vi "Open DSI.vi"(8 "error in (no error)":errorcluster, 11 "DCM":refnum<class "DCM - RT.lvclass">) -> (0 "error out":errorcluster, 2 "Target Name":string, 3 "DSI Reference":refnum<class "DCM-DSI.lvclass">)   [LabVIEW 2016, in "DCM-DSI.lvclass"]
uses:
  DCM-DSI.lvclass
  <vilib>/Powertrain Controls/Device Drivers/DCM/Rev0/RT/DCM - RT.lvclass
  <vilib>/Powertrain Controls/Device Drivers/DCM/Diff IO/RT/Results.ctl
  <vilib>/Powertrain Controls/Device Drivers/DCM/HH/RT/Config.ctl
  <vilib>/Powertrain Controls/Device Drivers/DCM/HH/RT/Mode.ctl
  <vilib>/Powertrain Controls/Device Drivers/DCM/HH/RT/ISeq.ctl
  <vilib>/Powertrain Controls/Device Drivers/DCM/HH/RT/Status.ctl
  <vilib>/Powertrain Controls/Device Drivers/DCM/Rev0/RT/System State.ctl
  <vilib>/Powertrain Controls/Device Drivers/DCM/Rev0/RT/System ADC.ctl
  <vilib>/Powertrain Controls/Device Drivers/DCM/Rev0/RT/Internal Fault.ctl
  <vilib>/Powertrain Controls/Device Drivers/Engine Position Tracking/EPTx/RevA/RT/Controls/EPTxData.ctl
  Shared/Typedefs/Engine-Channel.ctl
  DCM-DSI.lvclass/DCM-DSI.ctl
  <vilib>/addons/Software Calibration Management/xSCM/CalPoint.xnode
  <vilib>/Powertrain Controls/Device Drivers/DCM/Diff IO/RT/DCM - RT - Diff IO.lvlib
  <vilib>/Powertrain Controls/Device Drivers/DCM/HH/RT/DCM - RT - HH.lvlib
  <vilib>/Powertrain Controls/Device Drivers/Engine Position Tracking/EPTx/RevA/RT/EPTx - RevA - RT.lvlib
  <resource>/objmgr/nisysapi.rc
  <vilib>/NI_Real-Time Target Support.lvlib
  <vilib>/addons/Software Calibration Management/xSCM/ni_scm.dll
  Shared/DSI-Shared.lvlib
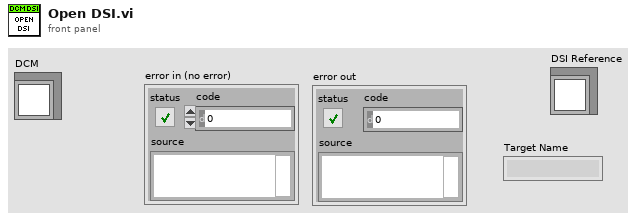
[diagram p1: front panel]
types:
  T1 = typedef "DSI-Shared.lvlib/Engine-Channel.ctl" = cluster{"Name":string, "Unit":string, "Value":sgl}
  T2 = typedef "EPTx - RevA - RT.lvlib/EPTxData.ctl" = cluster{"Sync":bool, "CurrentCAD":sgl, "Speed [RPM]":sgl, "Config":bool, "Rcvg Primary":bool, "Stall":bool, "Overflow":bool, "Ratio Error":bool, "Pattern Error":bool, "Aux Warning":bool, "Watchdog Error":bool}
  T3 = typedef "DCM - RT.lvclass/System State.ctl" = cluster{"System ADC":T4, "IO Lock":bool, "HH Mode Config Error":bool, "Fan Speed 1 [RPM]":sgl, "Fan Speed 2 [RPM]":sgl, "Firmware Major Rev":u16, "Firmware Minor Rev":u16, "Internal Fault":T5, "Fault Value":dbl}
  T4 = typedef "DCM - RT.lvclass/System ADC.ctl" = cluster{"AI 1 [V]":sgl, "AI 2 [V]":sgl, "AI 3 [V]":sgl, "AI 4 [V]":sgl, "AI 5 [V]":sgl, "AI 6 [V]":sgl, "AI 7 [V]":sgl, "AI 8 [V]":sgl, "AI 9 [V]":sgl, "AI 10 [V]":sgl, "AI 11 [V]":sgl, "AI 12 [V]":sgl, "Temp HH 1-6 [C]":sgl, "Temp HH 7-12 [C]":sgl, "Temp DI A [C]":sgl, "Temp DI Zener A [C]":sgl, "Temp DI B [C]":sgl, "Temp DI Zener B [C]":sgl, "Temp CPU [C]":sgl, "Temp Fan Intake [C]":sgl, "Temp Secondary A [C]":sgl, "Temp Primary A [C]":sgl, "Temp Boost B [C]":sgl, "Primary Range [V]":sgl, "Primary A1A2 [V]":sgl, "Primary A3A4 [V]":sgl, "Primary B3B4 [V]":sgl, "Primary B1B2 [V]":sgl, "Secondary A1A2 [V]":sgl, "Secondary A3A4 [V]":sgl, "Secondary B3B4 [V]":sgl, "Secondary B1B2 [V]":sgl, "Ext HV A [V]":sgl, "Ext HV B [V]":sgl, "FET Driver [V]":sgl, "Fan [V]":sgl, "Battery [V]":sgl, "DRVP [V]":sgl, "Key [V]":sgl, "DI Zener A [V]":sgl, "DI Zener B [V]":sgl, "Pump Zener A [V]":sgl, "Pump Zener B [V]":sgl, "MPRD [V]":sgl}
  T5 = typedef "DCM - RT.lvclass/Internal Fault.ctl" = enum32{"None", "Temp HH 1-6", "Temp HH 7-12", "Temp DI A", "Temp DI Zener A", "Temp DI B", "Temp DI Zener B", "Temp Intake", "Temp Primary A", "Temp Secondary A", "Temp Boost B", "Temp CPU", "Low Battery", "Inrush Protection", "A Run Enable", "B Run Enable", "Fan Speed"}
  T6 = typedef "DCM - RT - HH.lvlib/Status.ctl" = cluster{"Current [A]":sgl, "Config Error":bool, "Short Fault":bool, "Open Fault":bool, "Period Min [A]":sgl, "Period Max [A]":sgl, "Period Avg [A]":sgl, "On Avg [A]":sgl}
  T7 = typedef "DCM - RT - HH.lvlib/Config.ctl" = cluster{"Mode":T8, "IO Lock State":bool, "Phase 1 FP":bool, "Fault Clear":bool, "ISeq":T9[]}
  T8 = typedef "DCM - RT - HH.lvlib/Mode.ctl" = enum16{"Off", "Lowside", "Highside", "PFI", "Full H", "3-Phase"}
  T9 = typedef "DCM - RT - HH.lvlib/ISeq.ctl" = cluster{"Upper [A]":sgl, "Lower [A]":sgl, "Duration [s]":sgl}
  T10 = typedef "DCM - RT - Diff IO.lvlib/Results.ctl" = cluster{"Capture [DBTDC]":sgl, "Capture Error":bool, "Frequency [Hz]":sgl, "Duty Cycle [%]":sgl, "PWM Stopped":bool}
  T11 = cluster{"Mode":enum8{"Off", "Direct", "Calibration", "Triggered Multi-Pulse", "Engine Position Tracking"}, "Digital Input":enum8{"Unused", "User OS", "Diff IO 1", "Diff IO 2", "Diff IO 3", "Diff IO 4", "Diff IO 5", "Diff IO 6", "Diff IO 7", "Diff IO 8", "Aux 1", "Aux 2", "Aux 3", "Aux 4", "Aux 5", "Aux 6", "Aux 7", "Aux 8", "Aux 9", "Aux 10", "Aux 11", "Aux 12", "Aux 13", "Aux 14", "Aux 15", "Aux 16"}, "Default Profile Index":u8, "Cal Freq [Hz]":sgl, "Cal Duration [s]":sgl, "Cal Increment [s]":sgl, "Cal Pulses":u16, "TMP Command Sequence":cluster{"Duration [s]":sgl, "Level":bool, "Run/Stop":bool, "Profile Index":u8}[], "EPT TDC Offset [CAD]":sgl, "EPT Window Start [DBTDC]":sgl, "EPT Window End [DBTDC]":sgl, "EPT Angles":cluster{"Enable":bool, "Timing [DBTDC]":sgl, "Duration [s]":sgl, "Profile Index":u8}[], "EPT Skip Fire":bool, "EPT Skip Index":u8, "EPT Precharge Duration [s]":sgl, "EPT Precharge Profile Index":u8}[]
  T12 = cluster{"Mode":enum8{"Off", "Direct", "Calibration", "Triggered Multi-Pulse", "Engine Position Tracking"}, "Digital Input":enum8{"Unused", "User OS", "Diff IO 1", "Diff IO 2", "Diff IO 3", "Diff IO 4", "Diff IO 5", "Diff IO 6", "Diff IO 7", "Diff IO 8", "Aux 1", "Aux 2", "Aux 3", "Aux 4", "Aux 5", "Aux 6", "Aux 7", "Aux 8", "Aux 9", "Aux 10", "Aux 11", "Aux 12", "Aux 13", "Aux 14", "Aux 15", "Aux 16"}, "Default Profile Index":u8, "Cal Freq [Hz]":sgl, "Cal Duration [s]":sgl, "Cal Increment [s]":sgl, "Cal Pulses":u16, "TMP Command Sequence":cluster{"Duration [s]":sgl, "Level":bool, "Run/Stop":bool, "Profile Index":u8}[], "EPT TDC Offset [CAD]":sgl, "EPT Window Start [DBTDC]":sgl, "EPT Window End [DBTDC]":sgl, "EPT Angles":cluster{"Enable":bool, "Timing [DBTDC]":sgl, "Duration [s]":sgl, "Profile Index":u8}[], "EPT Skip Fire":bool, "EPT Skip Index":u8, "EPT Precharge Duration [s]":sgl, "EPT Precharge Profile Index":u8}
  T13 = cluster{"Mode":enum8{"Off", "Input", "Pulse Width Modulation", "Engine Position Tracking", "Serial Out 1", "Serial Out 2", "EPTx Sync"}, "Capture Start [DBTDC]":sgl, "Capture End [DBTDC]":sgl, "Invert":bool, "Frequency [Hz]":sgl, "Duty Cycle [%]":sgl, "TDC Offset [CAD]":sgl, "Window Start [DBTDC]":sgl, "Window End [DBTDC]":sgl, "Angles":cluster{"Enable":bool, "Location [DBTDC]":sgl, "Duration [s]":sgl}[], "Skip Fire":bool, "Skip Fire Index":u8}[]
  T14 = cluster{"Mode":enum8{"Off", "Direct", "Pulse Width Modulation", "Engine Position Tracking"}, "Digital Input":enum8{"Unused", "User OS", "Diff IO 1", "Diff IO 2", "Diff IO 3", "Diff IO 4", "Diff IO 5", "Diff IO 6", "Diff IO 7", "Diff IO 8", "Aux 1", "Aux 2", "Aux 3", "Aux 4", "Aux 5", "Aux 6", "Aux 7", "Aux 8", "Aux 9", "Aux 10", "Aux 11", "Aux 12", "Aux 13", "Aux 14", "Aux 15", "Aux 16"}, "Polarity":bool, "Frequency [Hz]":sgl, "Duty Cycle [%]":sgl, "TDC Offset [CAD]":sgl, "Window Start [DBTDC]":sgl, "Window End [DBTDC]":sgl, "Angles":cluster{"Enable":bool, "Location [DBTDC]":sgl, "Duration [s]":sgl}[], "Skip Fire":bool, "Skip Fire Index":u8}[]
  T15 = cluster{"Enable":bool, "Total Cycles":u8, "On Cycles":u8, "TDC Offset [CAD]":sgl}[]
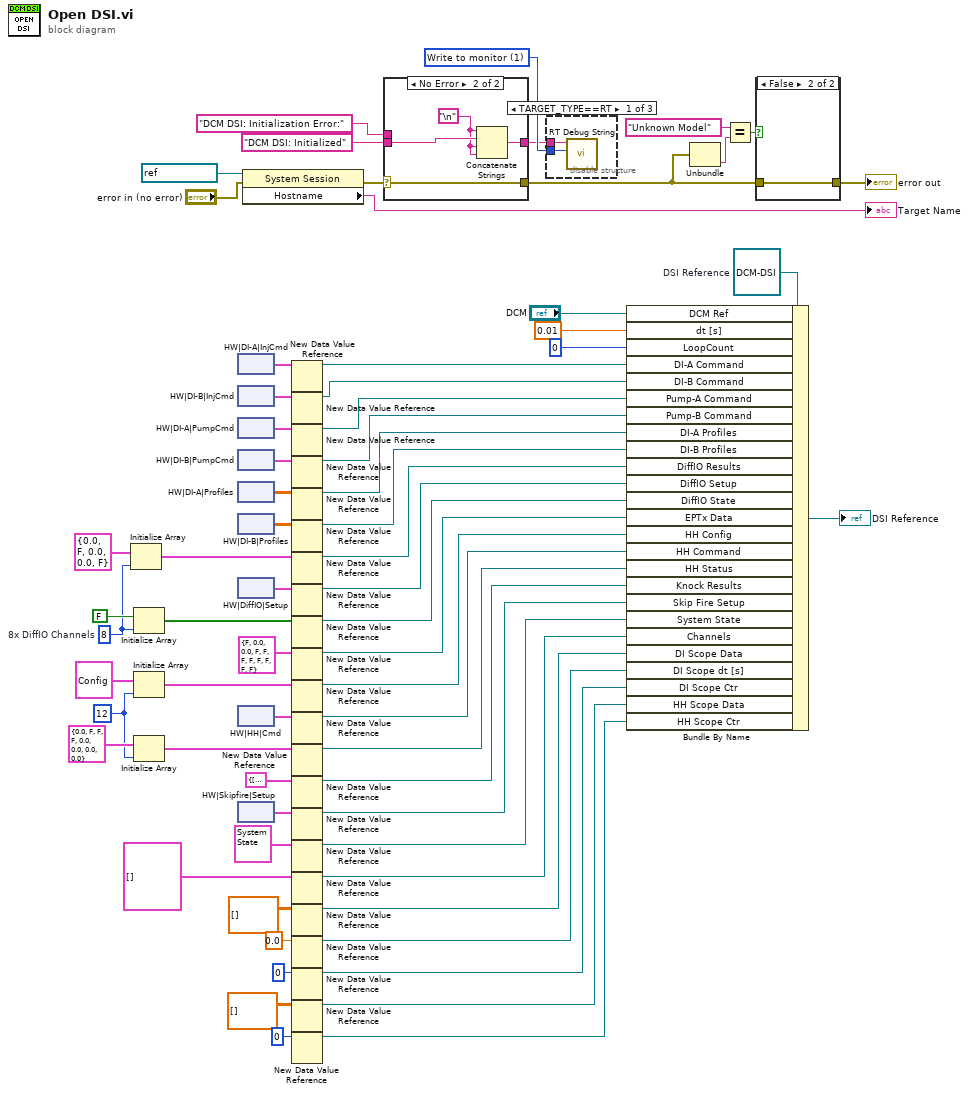
[diagram p0: block diagram]
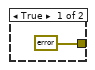
[diagram p4: hidden frame]
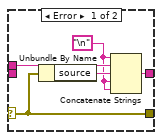
[diagram p5: hidden frame]
diagram:
  w10 = u16 1 items=["Write to serial", "Write to monitor", "Write to system log"] ("Interface")
  w56 = 12 ("dimension size")
  w19 = 8  # 8x DiffIO Channels
  w34 = refnum<class "DCM-DSI.lvclass"> refnum  # DSI Reference
  n1 = Initialize Array(T10 {"Capture [DBTDC]"=0.0, "Capture Error"=FALSE, "Frequency [Hz]"=0.0, "Duty Cycle [%]"=0.0, "PWM Stopped"=FALSE} ("Diff I/O Result"), w19) -> (w65:T10[])
  n2 = Initialize Array(FALSE ("Boolean"), w19) -> (w64:bool[])
  n3 = Initialize Array(T7 {"Mode"=enum."Off", "IO Lock State"=FALSE, "Phase 1 FP"=FALSE, "Fault Clear"=FALSE, "ISeq"=[{"Upper [A]"=0.0, "Lower [A]"=0.0, "Duration [s]"=0.0}, {"Upper [A]"=0.0, "Lower [A]"=0.0, "Duration [s]"=0.0}]} ("HH Config"), w56) -> (w62:T7[])
  n4 = Initialize Array(T6 {"Current [A]"=0.0, "Config Error"=FALSE, "Short Fault"=FALSE, "Open Fault"=FALSE, "Period Min [A]"=0.0, "Period Max [A]"=0.0, "Period Avg [A]"=0.0, "On Avg [A]"=0.0} ("HH Status"), w56) -> (w57:T6[])
  n5 = xnode "HW|DI-A|InjCmd"() -> ("Value"=w25:T11)
  n6 = xnode "HW|DI-B|InjCmd"() -> ("Value"=w23:T11)
  n7 = xnode "HW|DI-A|PumpCmd"() -> ("Value"=w24:T12)
  n8 = xnode "HW|DI-B|PumpCmd"() -> ("Value"=w22:T12)
  n9 = xnode "HW|DI-A|Profiles"() -> ("Value"=w21:sgl[][])
  n10 = xnode "HW|DI-B|Profiles"() -> ("Value"=w20:sgl[][])
  n11 = xnode "HW|DiffIO|Setup"() -> ("Value"=w17:T13)
  n12 = xnode "HW|HH|Cmd"() -> ("Value"=w16:T14)
  n13 = xnode "HW|Skipfire|Setup"() -> ("Value"=w15:T15)
  n14 = property class="System Session"(reference=refnum<k21> "localhost" ("Target (localhost)"), error in="error in (no error)") -> (error out=w1:errorcluster, "Hostname"=→"Target Name":string)  [unwired: 1 out]
  n15 = New Data Value Reference(data value=w25) -> (data value reference=w66:refnum<data-value>)  [unwired: 1 in, 1 out]
  n16 = New Data Value Reference(data value=w23) -> (data value reference=w26:refnum<data-value>)  [unwired: 1 in, 1 out]
  n17 = New Data Value Reference(data value=w24) -> (data value reference=w27:refnum<data-value>)  [unwired: 1 in, 1 out]
  n18 = New Data Value Reference(data value=w22) -> (data value reference=w28:refnum<data-value>)  [unwired: 1 in, 1 out]
  n19 = New Data Value Reference(data value=w21) -> (data value reference=w29:refnum<data-value>)  [unwired: 1 in, 1 out]
  n20 = New Data Value Reference(data value=w20) -> (data value reference=w30:refnum<data-value>)  [unwired: 1 in, 1 out]
  n21 = New Data Value Reference(data value=w65) -> (data value reference=w31:refnum<data-value>)  [unwired: 1 in, 1 out]
  n22 = New Data Value Reference(data value=w17) -> (data value reference=w18:refnum<data-value>)  [unwired: 1 in, 1 out]
  n23 = New Data Value Reference(data value=w64) -> (data value reference=w63:refnum<data-value>)  [unwired: 1 in, 1 out]
  n24 = New Data Value Reference(data value=T2 {"Sync"=FALSE, "CurrentCAD"=0.0, "Speed [RPM]"=0.0, "Config"=FALSE, "Rcvg Primary"=FALSE, "Stall"=FALSE, "Overflow"=FALSE, "Ratio Error"=FALSE, "Pattern Error"=FALSE, "Aux Warning"=FALSE, "Watchdog Error"=FALSE} ("HW.EPTxData")) -> (data value reference=w47:refnum<data-value>)  [unwired: 1 in, 1 out]
  n25 = New Data Value Reference(data value=w62) -> (data value reference=w60:refnum<data-value>)  [unwired: 1 in, 1 out]
  n26 = New Data Value Reference(data value=w16) -> (data value reference=w59:refnum<data-value>)  [unwired: 1 in, 1 out]
  n27 = New Data Value Reference(data value=w57) -> (data value reference=w55:refnum<data-value>)  [unwired: 1 in, 1 out]
  n28 = New Data Value Reference(data value=cluster{"Knock":bool[], "Knock Intensity":sgl[]} {"Knock"=[FALSE, FALSE, FALSE, FALSE, FALSE, FALSE, FALSE, FALSE, FALSE, FALSE, FALSE, FALSE, FALSE, FALSE, FALSE, FALSE], "Knock Intensity"=[0.0, 0.0, 0.0, 0.0, 0.0, 0.0, 0.0, 0.0, 0.0, 0.0, 0.0, 0.0, 0.0, 0.0, 0.0, 0.0]} ("HW.Knock Results")) -> (data value reference=w51:refnum<data-value>)  [unwired: 1 in, 1 out]
  n29 = New Data Value Reference(data value=w15) -> (data value reference=w54:refnum<data-value>)  [unwired: 1 in, 1 out]
  n30 = New Data Value Reference(data value=T3 {"System ADC"={"AI 1 [V]"=0.0, "AI 2 [V]"=0.0, "AI 3 [V]"=0.0, "AI 4 [V]"=0.0, "AI 5 [V]"=0.0, "AI 6 [V]"=0.0, "AI 7 [V]"=0.0, "AI 8 [V]"=0.0, "AI 9 [V]"=0.0, "AI 10 [V]"=0.0, "AI 11 [V]"=0.0, "AI 12 [V]"=0.0, "Temp HH 1-6 [C]"=0.0, "Temp HH 7-12 [C]"=0.0, "Temp DI A [C]"=0.0, "Temp DI Zener A [C]"=0.0, "Temp DI B [C]"=0.0, "Temp DI Zener B [C]"=0.0, "Temp CPU [C]"=0.0, "Temp Fan Intake [C]"=0.0, "Temp Secondary A [C]"=0.0, "Temp Primary A [C]"=0.0, "Temp Boost B [C]"=0.0, "Primary Range [V]"=0.0, "Primary A1A2 [V]"=0.0, "Primary A3A4 [V]"=0.0, "Primary B3B4 [V]"=0.0, "Primary B1B2 [V]"=0.0, "Secondary A1A2 [V]"=0.0, "Secondary A3A4 [V]"=0.0, "Secondary B3B4 [V]"=0.0, "Secondary B1B2 [V]"=0.0, "Ext HV A [V]"=0.0, "Ext HV B [V]"=0.0, "FET Driver [V]"=0.0, "Fan [V]"=0.0, "Battery [V]"=0.0, "DRVP [V]"=0.0, "Key [V]"=0.0, "DI Zener A [V]"=0.0, "DI Zener B [V]"=0.0, "Pump Zener A [V]"=0.0, "Pump Zener B [V]"=0.0, "MPRD [V]"=0.0}, "IO Lock"=FALSE, "HH Mode Config Error"=FALSE, "Fan Speed 1 [RPM]"=0.0, "Fan Speed 2 [RPM]"=0.0, "Firmware Major Rev"=0, "Firmware Minor Rev"=0, "Internal Fault"=enum."None", "Fault Value"=0.0} ("System State")) -> (data value reference=w52:refnum<data-value>)  [unwired: 1 in, 1 out]
  n31 = New Data Value Reference(data value=T1[] [] ("ENG.Channel")) -> (data value reference=w46:refnum<data-value>)  [unwired: 1 in, 1 out]
  n32 = New Data Value Reference(data value=sgl[][] []) -> (data value reference=w45:refnum<data-value>)  [unwired: 1 in, 1 out]
  n33 = New Data Value Reference(data value=sgl 0.0) -> (data value reference=w44:refnum<data-value>)  [unwired: 1 in, 1 out]
  n34 = New Data Value Reference(data value=u32 0 ("dimension size")) -> (data value reference=w43:refnum<data-value>)  [unwired: 1 in, 1 out]
  n35 = New Data Value Reference(data value=sgl[][] []) -> (data value reference=w42:refnum<data-value>)  [unwired: 1 in, 1 out]
  n36 = New Data Value Reference(data value=u32 0 ("dimension size")) -> (data value reference=w41:refnum<data-value>)  [unwired: 1 in, 1 out]
  n37 = case shown="No Error" w1 {
    selector: w1 -> [w69 w77]
    tunnel: [w69 w77] -> w4
    tunnel: "DCM DSI: Initialization Error:" ("String to write") -> [w73 _]
    tunnel: "DCM DSI: Initialized" ("String to write") -> [_ w76]
    tunnel: [w70 w74] -> w9
    frame Error {
      w71 = "\n"
      n38 = Unbundle By Name(w69) -> ("source"=w72:string)
      n39 = Concatenate Strings(w71, w73, w72, w71, w71) -> (w70:string)
    }
    frame No Error {
      w75 = "\n"
      n40 = Concatenate Strings(w75, w76, w75, w75) -> (w74:string)
    }
  }
  n41 = disable-structure shown="TARGET_TYPE==RT" {
    disable-tunnel: w10 -> [w79 _ _]
    disable-tunnel: w9 -> [w78 _ _]
    frame condition #0 (active) {
      n42 = call <vilib>:"RT Debug String.vi"("Interface"=w79, "String to write"=w78) -> ()  [unwired: 9 in, 1 out]
    }
    frame condition #1 {
    }
    frame condition #2 {
    }
  }
  n43 = Bundle By Name(cluster=w34, "DCM Ref"="DCM", "dt [s]"=0.01 ("Numeric"), "LoopCount"=0, "DI-A Command"=w66, "DI-B Command"=w26, "Pump-A Command"=w27, "Pump-B Command"=w28, "DI-A Profiles"=w29, "DI-B Profiles"=w30, "DiffIO Results"=w31, "DiffIO Setup"=w18, "DiffIO State"=w63, "EPTx Data"=w47, "HH Config"=w60, "HH Command"=w59, "HH Status"=w55, "Knock Results"=w51, "Skip Fire Setup"=w54, "System State"=w52, "Channels"=w46, "DI Scope Data"=w45, "DI Scope dt [s]"=w44, "DI Scope Ctr"=w43, "HH Scope Data"=w42, "HH Scope Ctr"=w41) -> (→"DSI Reference":refnum<class "DCM-DSI.lvclass">)
  n44 = Unbundle(w4) -> ("source"=w7:string)  [unwired: 2 out]
  n45 = Equal?(x="Unknown Model", y=w7) -> (x = y?=w5:bool)
  n46 = case shown="False" w5 {
    tunnel: [errorcluster {"status"=FALSE, "code"=0, "source"=""} ("error IO") w81] -> w8
    tunnel: w4 -> [_ w81]
    frame True {
    }
    frame False {
    }
  }
  "error out" <- w8
